vi "post_experiment_settings.vi"(8 "error in (no error)":errorcluster, 10 "Small?":bool, 11 "Cluster":T1) -> (0 "error out":errorcluster)   [LabVIEW 2013]
doc: "Adds a the given cluster to the pelletron_data table."
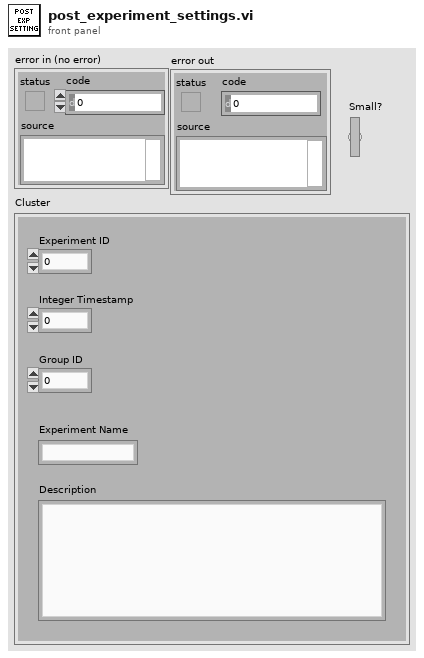
[diagram p1: front panel]
types:
  T1 = cluster{"Experiment ID":i32, "Integer Timestamp":i64, "Group ID":u16, "Experiment Name":string, "Description":string}
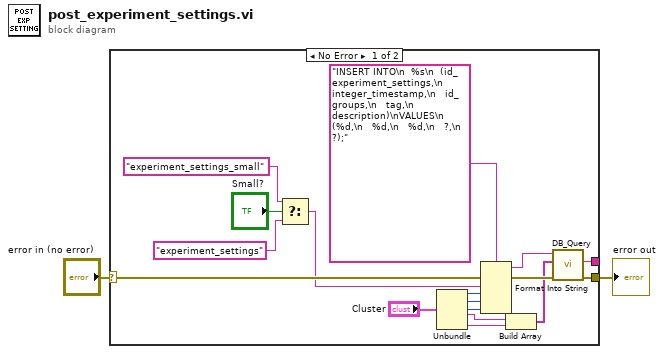
[diagram p0: block diagram]
diagram:
  n1 = case shown="No Error" "error in (no error)" {
    selector: "error in (no error)" -> [w15 w20]
    tunnel: [w7 w20] -> w1
    tunnel: [w6 _] -> _
    frame No Error {
      n2 = Select(t="experiment_settings_small", s="Small?", f="experiment_settings") -> (s? t:f=w12:string)
      n3 = Unbundle("Cluster") -> ("Experiment ID"=w10:i32, "Integer Timestamp"=w9:i64, "Group ID"=w8:u16, "Experiment Name"=w5:string, "Description"=w4:string)
      n4 = Format Into String(format string="INSERT INTO\n  %s\n  (id_experiment_settings,\n   integer_timestamp,\n   id_groups,\n   tag,\n   description)\nVALUES\n  (%d,\n   %d,\n   %d,\n   ?,\n   ?);" ("Parameterized Query"), error in=w15, w12, w10, w9, w8) -> (resulting string=w14:string, error out=w16:errorcluster)  [unwired: 1 in]
      n5 = Build Array(w5, w4) -> (w3:string[])
      n6 = call "DB_Query.vi"("error in (no error)"=w16, "Parameters"=w3, "Parameterized Query"=w14) -> ("error out"=w7:errorcluster, "Query in Standard Format"=w6:string)  [unwired: 6 in, 1 out]
    }
    frame Error {
    }
  }
  "error out" <- w1
